vi "BME_DG_ReadParameterFile_mittels array.vi"(8 "error in (no error)":errorcluster, 11 "Path":path=path "C:/Dokumente und Einstellungen/A2.5/Desktop/POLARIS BME DG/ParameterFiles/20120327 mit StandAloneAppl von 20120323.g0y") -> (0 "error out":errorcluster, 1 "Slave or Master":T3[](array[typedef]), 3 "#DGs":i32, 4 "CalibrateTiming":u32, 5 "CalibrationLevel":u32)   [LabVIEW 2009]
uses:
  BME_DG_MasterOrSlave.ctl
  Typedefs For ReadParameters()/BME_DG_BME_State.ctl
  Typedefs For ReadParameters()/BME_DG_DelayChannelData.ctl
  Typedefs For ReadParameters()/BME_DG_State_V2.ctl
  Typedefs For ReadParameters()/BME_DG_BME_Control_V2.ctl
  Typedefs For ReadParameters()/BME_DG_DelayChannelData_V2.ctl
  Typedefs For ReadParameters()/BME_DG_DelayTriggerData_V2.ctl
  BME DLL/DelayGenerator.dll
panel:
  out "DGS":u8[](array[numeric])
  out "State":T1
  in  "p_CalibrationLevel":u32
  in  "p_CalibrateTiming":u32
  in  "#DG in":i32
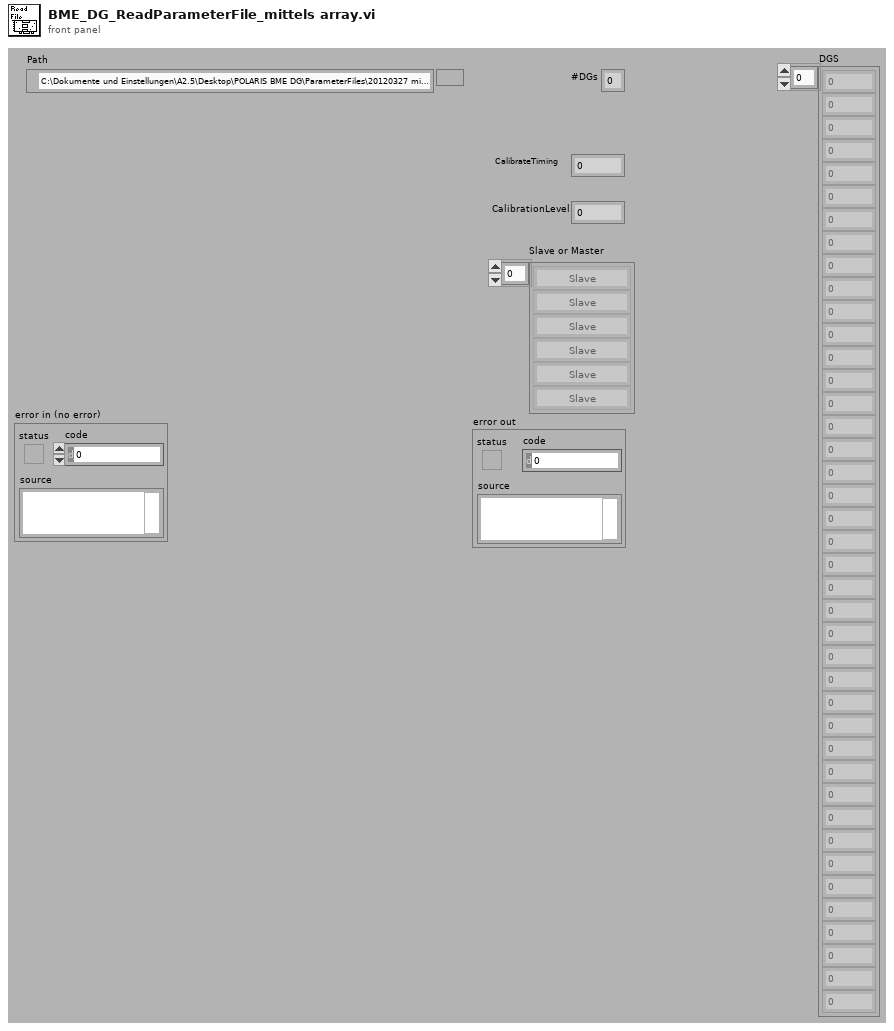
[diagram p1: front panel]
types:
  T1 = typedef "BME_DG_BME_State.ctl" = cluster{"T0":T2, "A":T2, "B":T2, "DT":cluster{"dTriggerLevel":dbl, "dInternalClock or dInhibitTrigger":dbl, "dForceTrigger":dbl, "ulPresetValue":u32, "ulDivideBy or sOscillatorDivider+sTriggerDivider":u32, "ulClockSource":u32, "ulGateDivider":u32, "ulMS_Bus":u32, "bPositiveGate":u32, "bIgnoreGate":u32, "bSynchronizeGate":u32, "bClockEnable":u32, "bInternalTrigger":u32, "bInternalArm":u32, "bSoftwareTrigger":u32, "bRisingEdge":u32, "bStopOnPreset":u32, "bResetWhenDone":u32, "bTriggerEnable":u32, "bTerminate":u32, "bReserve":u32}, "bGate_AB":u32, "ulGateFunction":u32, "ulOuputLevel":u32, "ulDG_Product":u32, "ulPulseWidth":u32, "fill int 1":i32, "fill int 2":i32, "fill int 3":i32, "fill int 4":i32, "fill int 5":i32}
  T2 = typedef "BME_DG_DelayChannelData.ctl" = cluster{"FireFirst":dbl, "SetBack":dbl, "FireSecond":dbl, "OutputModulo":u32, "OutputOffset":u32, "GoSignal":u32, "DoneSignal":u32, "bPositive":u32, "bTerminate":u32, "bHighDrive":u32, "bReserve":u32}
  T3 = typedef "BME_DG_MasterOrSlave.ctl" = enum16{"Unknown", "Master", "Slave"}
  T4 = typedef "BME_DG_State_V2.ctl" = cluster{"Control":T5, "lBaseAddress":i32, "lDG_Produkt":i32, "bMaster":u32, "lBusNumber":i32, "strIPAddress":string}
  T5 = typedef "BME_DG_BME_Control_V2.ctl" = cluster{"T0":T6, "A":T6, "B":T6, "C":T6, "D":T6, "E":T6, "F":T6, "DelayTrigger":T7, "bGate_AB":u32, "ulGateFunction":u32, "ulOuputLevel":u32, "ulPulseWidth":u32}
  T6 = typedef "BME_DG_DelayChannelData_V2.ctl" = cluster{"DelayTimes":dbl[], "PulseWidths":dbl[], "SetBack":dbl, "StepsBack":u32[], "ListLength":i32, "OutputModulo":u32, "OutputOffset":u32, "GoSignal":u32, "DoneSignal":u32, "bPositive":u32, "bTerminate":u32, "bHighDrive":u32, "bDisconnect":u32, "bOntoMsBus":u32, "bInputPositive":u32}
  T7 = typedef "BME_DG_DelayTriggerData_V2.ctl" = cluster{"dTriggerLevel":dbl, "dGateLevel":dbl, "dInternalClock or dInhibitTrigger":dbl, "dInhibitSecondary":dbl, "dForceTrigger":dbl, "dStepBackTime":dbl, "dGateDelay":dbl, "ulBurstCounter":u32, "ulDelaySecundary":u32, "l64Preset Value":i64, "ulDivideBy or sOscillatorDivider+sTriggerDivider":u32, "ulTriggerMuliplier":u32, "ulClockSource":u32, "ulGateDivider":u32, "ulMS_Bus":u32, "bPositiveGate":u32, "bIgnoreGate":u32, "bSynchronizeGate":u32, "bClockEnable":u32, "bInternalTrigger":u32, "bInternalArm":u32, "bSoftwareTrigger":u32, "bRisingEdge":u32, "bStopOnPreset":u32, "bResetWhenDone":u32, "bTriggerEnable":u32, "bTerminate":u32, "bUseF":u32}
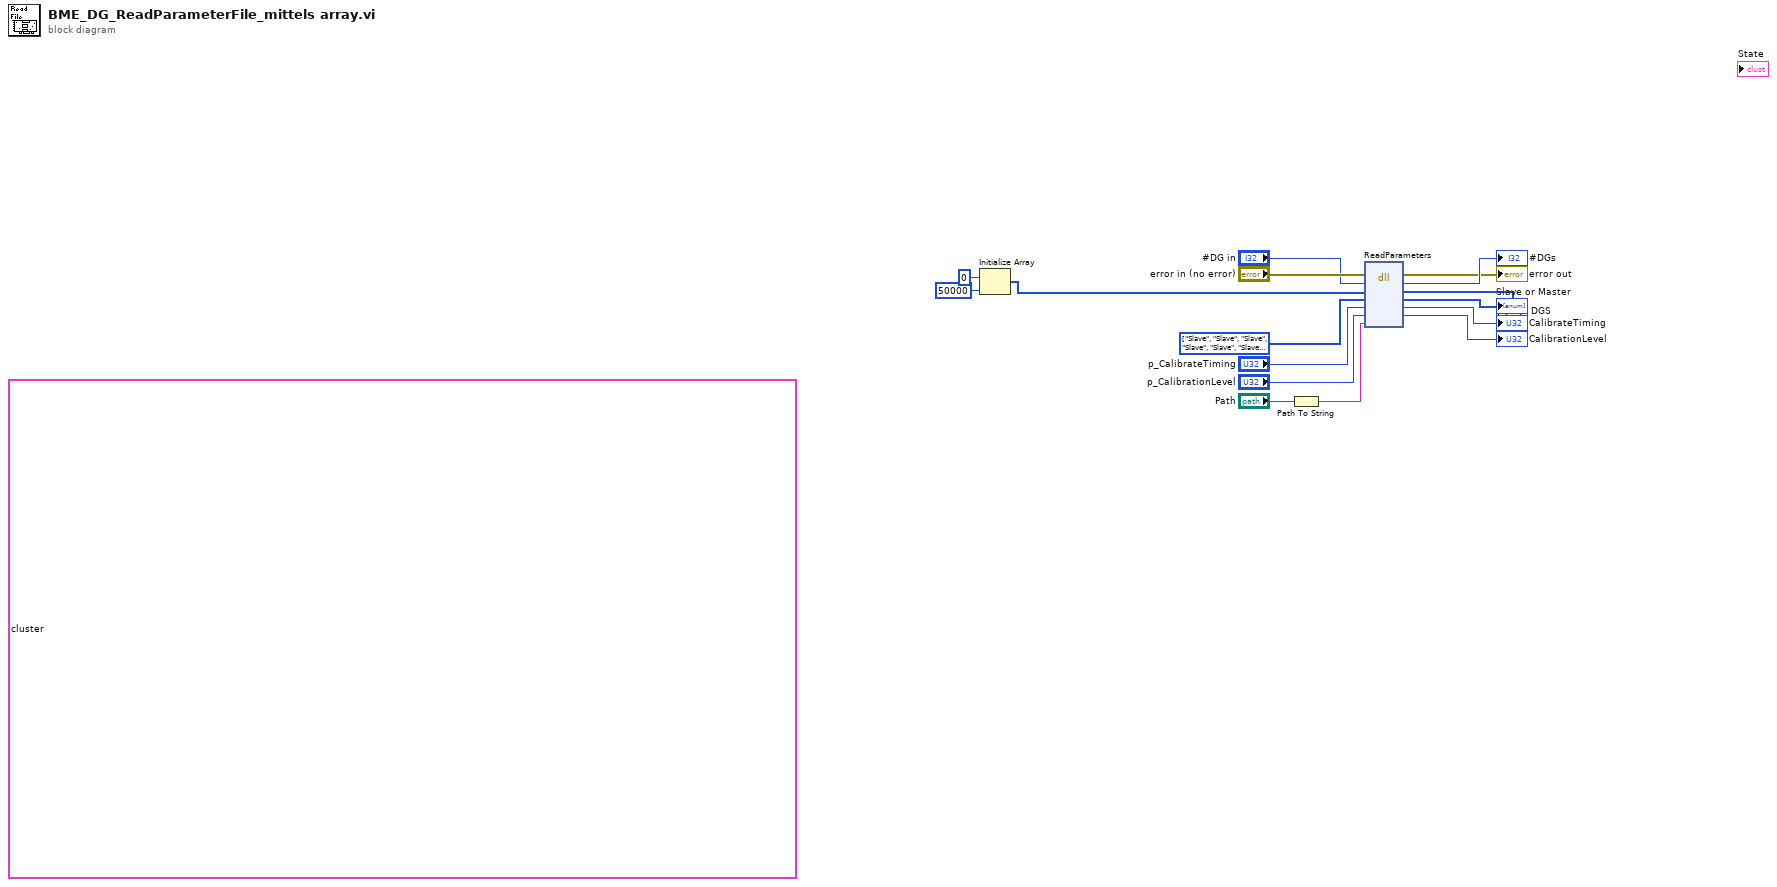
[diagram p0: block diagram]
diagram:
  (unwired) cluster{"BME_DG_BME_State":T4} data[72348B]
  w5 = T3[] [enum."Slave", enum."Slave", enum."Slave", enum."Slave", enum."Slave", enum."Slave", enum."Slave", enum."Slave", enum."Slave", enum."Slave", enum."Slave", enum."Slave", enum."Slave", enum."Slave", enum."Slave", enum."Slave", enum."Slave", enum."Slave", enum."Slave", enum."Slave", enum."Slave", enum."Slave", enum."Slave", enum."Slave", enum."Slave", enum."Slave", enum."Slave", enum."Slave", enum."Slave", enum."Slave", enum."Slave", enum."Slave", enum."Slave", enum."Slave", enum."Slave", enum."Slave", enum."Slave", enum."Slave", enum."Slave", enum."Slave", enum."Slave", enum."Slave", enum."Slave", enum."Slave", enum."Slave", enum."Slave", enum."Slave", enum."Slave", enum."Slave", enum."Slave", enum."Unknown"] items=["Unknown", "Master", "Slave"]
  n1 = Initialize Array(u8 0 ("element"), 50000 ("dimension size")) -> (w2:u8[])
  n2 = Path To String(path="Path") -> (string=w12:string)
  n3 = dll-call lib="C:/Dokumente und Einstellungen/A2.5/Desktop/POLARIS BME DG/BME DLL/DelayGenerator.dll" fn="ReadParameters" label="Activate_DG_BME"(error in="error in (no error)", "#DG"="#DG in", "DGS"=w2, "module"=w5, "CalibrateTiming"="p_CalibrateTiming", "CalibrationLevel"="p_CalibrationLevel", "FileName"=w12) -> (error out=→"error out":errorcluster, "#DG"=→"#DGs":i32, "DGS"=→"DGS":u8[], "module"=→"Slave or Master":i32[], "CalibrateTiming"=→"CalibrateTiming":u32, "CalibrationLevel"=→"CalibrationLevel":u32)  [unwired: 2 in, 1 out]
